vi "Memory.Pointer.Bounds Check.Offset.vi"(8 "error in (no error)":errorcluster, 10 "offset":i64 format="%d bytes", 11 "Pointer in":refnum<class "Memory.Pointer.lvclass">) -> (0 "error out":errorcluster, 1 "offset valid":bool, 2 "offset out":i64 format="%d bytes", 3 "Pointer out":refnum<class "Memory.Pointer.lvclass">)   [LabVIEW 2016, in "LabVIEW Memory Manager.lvlib" / "Memory.Pointer.lvclass"]
uses:
  Memory.Pointer.lvclass
  Memory.Pointer.lvclass/Memory.Pointer.ctl
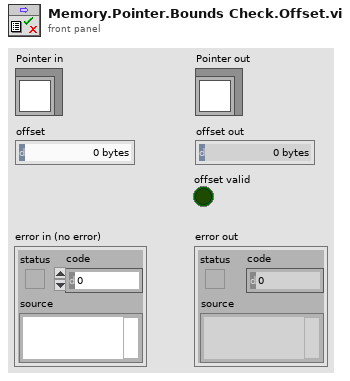
[diagram p1: front panel]
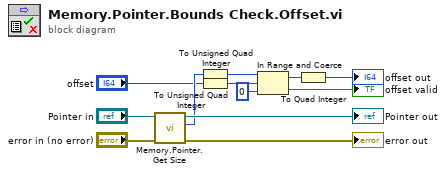
[diagram p0: block diagram]
diagram:
  n1 = call "Memory.Pointer.Get Size.vi"("error in (no error)"="error in (no error)", "Pointer in"="Pointer in") -> ("error out"=→"error out":errorcluster, "size"=w5:i64, "Pointer out"=→"Pointer out":refnum<class "Memory.Pointer.lvclass">)  [unwired: 7 in]
  n2 = To Unsigned Quad Integer(1:w5) -> (0:w11:u64)
  n3 = To Unsigned Quad Integer(1:"offset") -> (0:w10:u64)
  n4 = In Range and Coerce(upper limit=w11, x=w10, lower limit=u64 0) -> (coerced(x)=w3:u64, In Range?=→"offset valid":bool)
  n5 = To Quad Integer(1:w3) -> (0:→"offset out":i64)
